vi "Event Loop.vi"(11 "Hello World Event in":refnum<class "Hello World Event.lvclass">) -> (3 "Hello World Event out":refnum<class "Hello World Event.lvclass">)   [LabVIEW 2021, in "Hello World Event.lvlib" / "Hello World Event.lvclass"]
uses:
  Hello World Event.lvclass
  C:/git/jettl/src/Actor/Actor/Actor.lvclass
  Hello World Event.lvclass/Hello World Event.ctl
  Actor/Msgs/Teardown/Teardown Msg/Teardown Msg.lvclass
  C:/git/jettl/src/Actor/Msg/Msg.lvclass
  Actor/Event Actor/Event Actor.lvclass
  Actor/Msg/Msg.lvclass
panel:
  out "String Indicator":string
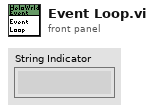
[diagram p1: front panel]
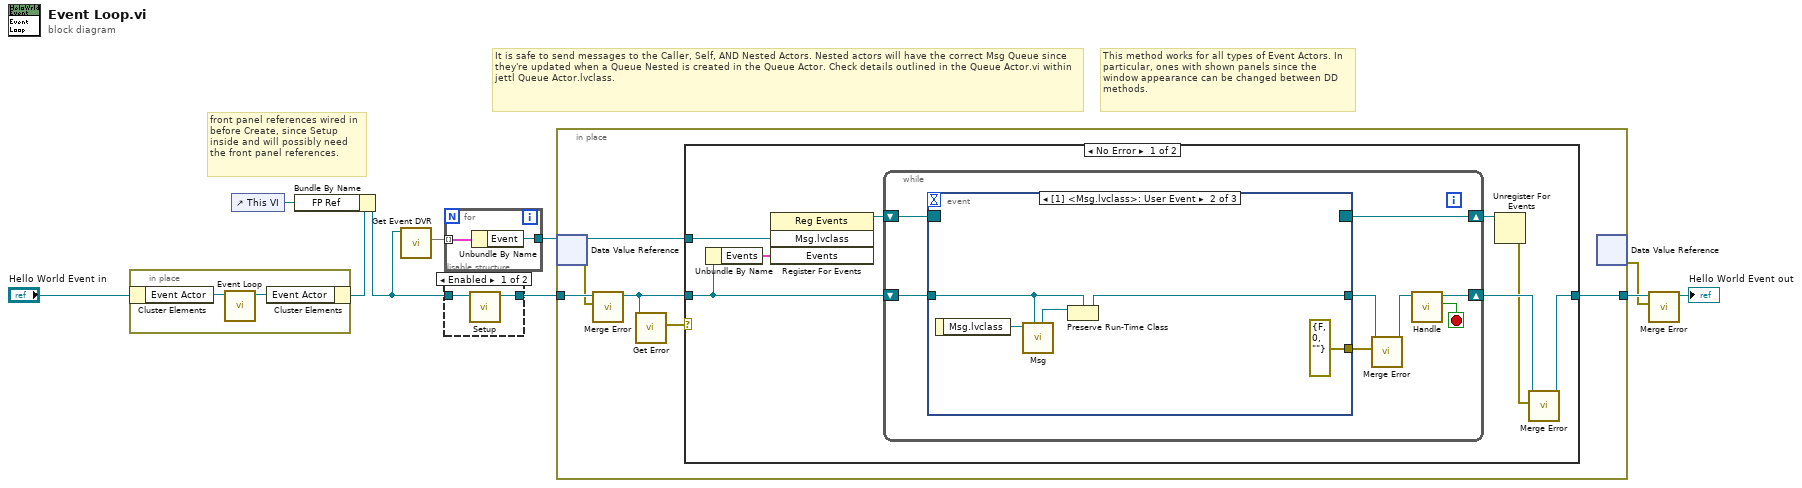
[diagram p0: block diagram]
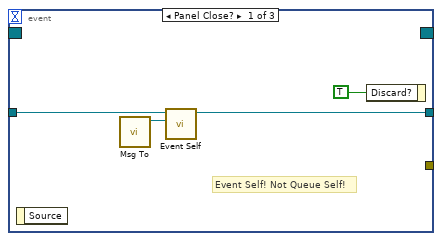
[diagram p3: hidden frame]
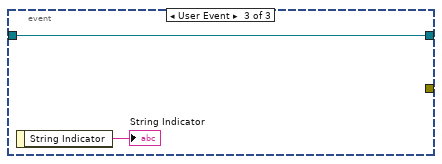
[diagram p4: hidden frame]
diagram:
  # "front panel references wired in before Create, since Setup inside and will possibly need the front panel references."
  # "This method works for all types of Event Actors. In particular, ones with shown panels since the window appearance can be changed between DD methods."
  # "It is safe to send messages to the Caller, Self, AND Nested Actors. Nested actors will have the correct Msg Queue since they're updated when a Queue Nested is created in the Queue Actor. Check details outlined in the Queue Actor.vi within jettl Queue Actor.lvclass."
  n1 = in-place {
    n2 = in-place-cluster #1("Hello World Event in") -> ("Event Actor"=w12:refnum<class "Event Actor.lvclass">)
    n3 = call-dynamic "Event Loop.vi"("Event Actor in"=w12) -> ("Event Actor out"=w11:refnum<class "Event Actor.lvclass">)  [unwired: 10 in]
    n4 = in-place-cluster #1("Event Actor"=w11) -> (w9:refnum<class "Hello World Event.lvclass">)
  }
  n5 = control-ref of="This VI"() -> (w1:refnum<vi>)
  n6 = Bundle By Name(cluster=w9, "FP Ref"=w1) -> (w3:refnum<class "Hello World Event.lvclass">)
  n7 = call-dynamic "Get Event DVR.vi"("Hello World Event in"=w3) -> ("Event Self"=w8:map{string, refnum<data-value>})  [unwired: 10 in]
  n8 = for {
    tunnel: w8 -> [w14] mode=indexing
    tunnel: [w13] -> w7
    n9 = Unbundle By Name(w14) -> ("Event"=w13:refnum<data-value>)
  }
  n10 = disable-structure shown="Enabled" {
    disable-tunnel: w3 -> [w16 w17]
    disable-tunnel: [w15 w17] -> w2
    frame Enabled {
      n11 = call-dynamic "Setup.vi"("Hello World Event in"=w16) -> ("Hello World Event out"=w15:refnum<class "Hello World Event.lvclass">)  [unwired: 10 in]
    }
    frame Disabled {
    }
  }
  n12 = in-place {
    in-place-border: w2 -> [w21]
    in-place-border: [w22] -> w6
    n13 = in-place-dvr #2(w7) -> (w23:refnum<user-event>, w20:errorcluster)
    n14 = call-dynamic "Merge Error.vi"("Error"=w20, "Set Error in"=w21) -> ("Set Error out"=w18:refnum<class "Hello World Event.lvclass">)  [unwired: 9 in]
    n15 = call-dynamic "Get Error.vi"("Hello World Event in"=w18) -> ("Error"=w19:errorcluster)  [unwired: 10 in]
    n16 = case shown="No Error" w19 {
      tunnel: w23 -> [w28 _]
      tunnel: [w25 w51] -> w22
      tunnel: w18 -> [w24 w51]
      frame No Error {
        n17 = Unbundle By Name(w24) -> ("Events"=w29:cluster{"String Indicator":refnum<user-event>})
        n18 = register-events ("Main Register for Events")(w28, w29) -> (reference out=w30:refnum<event-registration>)  [unwired: 2 in, 1 out]
        n19 = while {
          shift-right: [w35] -> w27
          shift-left: w24 -> [w37]
          shift-right: [w38] -> w31
          shift-left: w30 -> [w39]
          stop <- w34 stop-if-true
          n20 = event "UI Events" shown="[1] <Msg.lvclass>: User Event" {
            selector: w39 -> [_ _ _]
            dyn-events: [_ _ _] -> w38
            timeout: _ -> [_ _ _]
            tunnel: [w41 w46 w50] -> w32
            tunnel: w37 -> [w42 w48 w50]
            tunnel: [_ errorcluster {"status"=FALSE, "code"=0, "source"=""} ("error out") _] -> w36
            event Panel Close? {
              # "Event Self! Not Queue Self!"
              n21 = event-data() -> ()  [unwired: 1 in, 1 out]
              n22 = call "Msg To.vi"() -> ("Teardown Msg out"=w40:refnum<class "Teardown Msg.lvclass">)  [unwired: 11 in]
              n23 = call-dynamic "Event Self.vi"("Msg"=w40, "Hello World Event in"=w42) -> ("Hello World Event out"=w41:refnum<class "Hello World Event.lvclass">)  [unwired: 9 in]
              n24 = event-data("Discard?"=TRUE) -> ()  [unwired: 1 in, 1 out]
            }
            event User Event {
              n25 = event-data() -> ("Msg.lvclass"=w44:refnum<class "Msg.lvclass">)  [unwired: 1 in]
              n26 = call-dynamic "Msg.vi"("Actor in"=w48, "Msg in"=w44) -> ("Actor out"=w47:refnum<class "Actor.lvclass">)  [unwired: 9 in]
              n27 = Preserve Run-Time Class(object in=w47, 2:w48) -> (object out=w46:refnum<class "Hello World Event.lvclass">)  [unwired: 1 in, 1 out]
            }
            event User Event {
              n28 = event-data() -> ("String Indicator"=→"String Indicator":string)  [unwired: 1 in]
            }
          }
          n29 = call-dynamic "Merge Error.vi"("Error"=w36, "Set Error in"=w32) -> ("Set Error out"=w33:refnum<class "Hello World Event.lvclass">)  [unwired: 9 in]
          n30 = call-dynamic "Handle.vi"("Hello World Event in"=w33) -> ("Destroy?"=w34:bool, "Hello World Event out"=w35:refnum<class "Hello World Event.lvclass">)  [unwired: 9 in]
        }
        n31 = Unregister For Events(event registration refnum=w31) -> (error out=w26:errorcluster)  [unwired: 1 in]
        n32 = call-dynamic "Merge Error.vi"("Error"=w26, "Set Error in"=w27) -> ("Set Error out"=w25:refnum<class "Hello World Event.lvclass">)  [unwired: 9 in]
      }
      frame Error {
      }
    }
    n33 = in-place-dvr #2() -> (w4:errorcluster)  [unwired: 1 in, 1 out]
  }
  n34 = call-dynamic "Merge Error.vi"("Error"=w4, "Set Error in"=w6) -> ("Set Error out"=→"Hello World Event out":refnum<class "Hello World Event.lvclass">)  [unwired: 9 in]
